vi "PH_ImageCalibrator.read calibration data.vi"(2 "Calibration Data File":path, 5 "error in (no error)":errorcluster) -> (17 "Calibration data":T1, 19 "error out":errorcluster)   [LabVIEW 2014, in "PH_ImageCalibrator.lvlib"]
doc: "This VI reads out the calibration data file. If error in shows an error, the error is passing throung and nothing is done. If there is no incoming error, but an error ocours opening the file, reading the file or unpacking the data, error out is cleaned and the calibration data array is set to be empty. Otherwise the data are given out at the Calibration data cluster."
uses:
  PH_ImageCalibrator.lvlib
  PH_ImageCalibrator.Calibration Data.ctl
  PH_ImageCalibrator.Calibration Data - Version 1.ctl
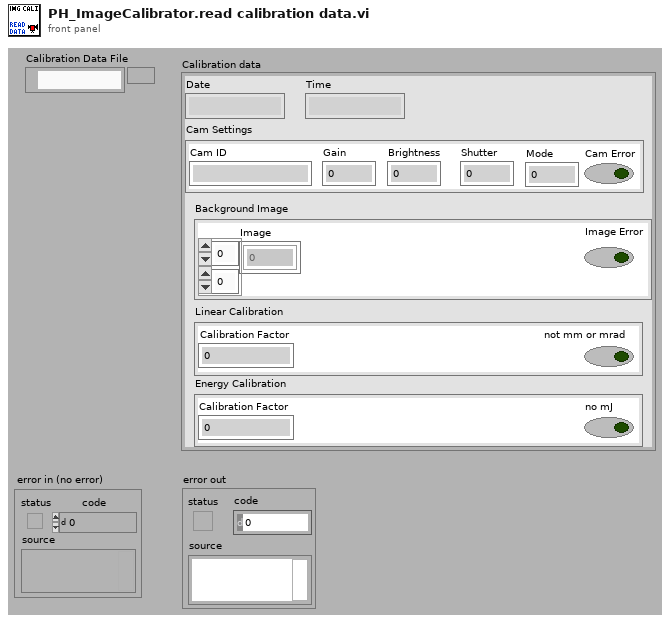
[diagram p1: front panel]
types:
  T1 = typedef "PH_ImageCalibrator.lvlib/PH_ImageCalibrator.Calibration Data.ctl" = cluster{"Date":string, "Time":string, "Cam Settings":cluster{"Cam ID":string, "Gain":dbl, "Brightness":dbl, "Shutter":dbl, "Cam Error":bool, "Mode":i32}, "Background Image":cluster{"Image":dbl[][], "Image Error":bool}, "Linear Calibration":cluster{"Calibration Factor":dbl, "not mm or mrad":bool}, "Energy Calibration":cluster{"Calibration Factor":dbl, "no mJ":bool}}
  T2 = typedef "PH_ImageCalibrator.lvlib/PH_ImageCalibrator.Calibration Data - Version 1.ctl" = cluster{"Date":string, "Time":string, "Cam Settings":cluster{"Serial Number":dbl, "Gain":i32, "Brightness":i32, "Shutter":i32, "Cam Error":bool, "Mode":i32}, "Background Image":cluster{"Image":dbl[][], "Image Error":bool}, "Linear Calibration":cluster{"Calibration Factor":dbl, "not mm or mrad":bool}, "Energy Calibration":cluster{"Calibration Factor":dbl, "no mJ":bool}}
  T3 = cluster{"Calibration Factor":dbl, "not mm or mrad":bool}
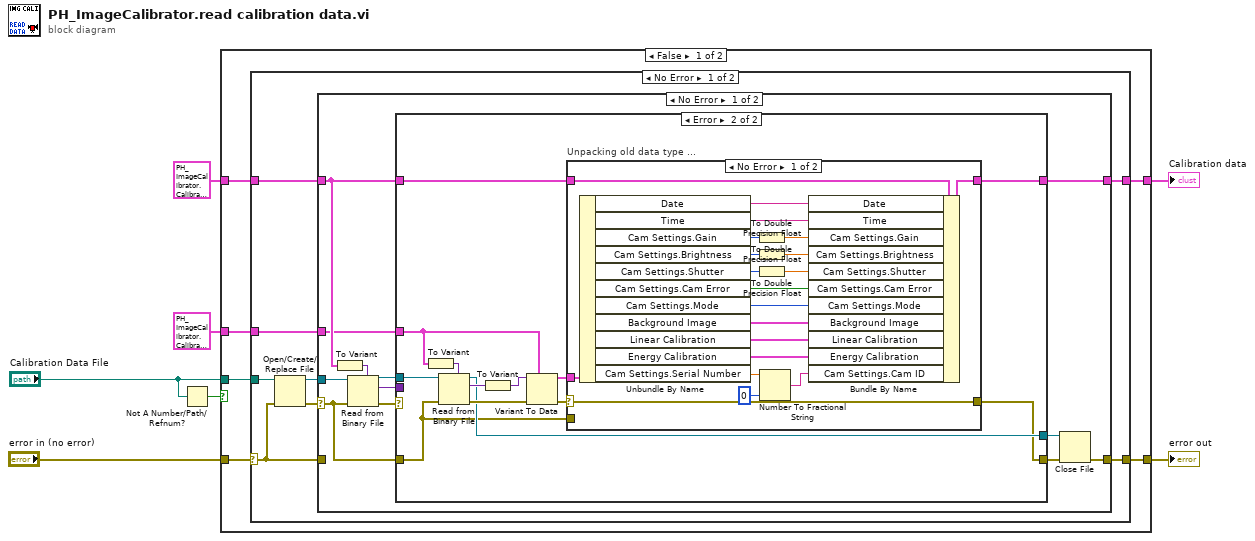
[diagram p0: block diagram]
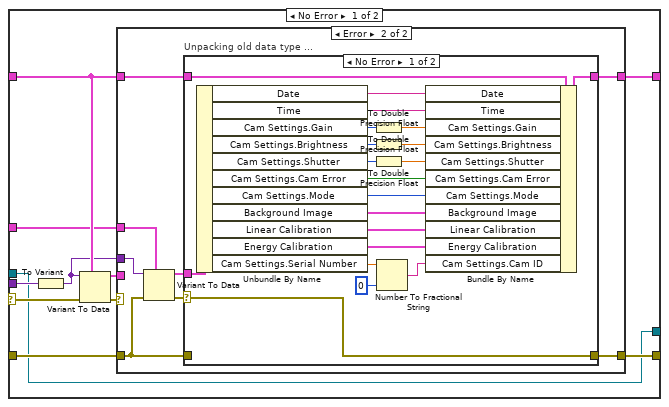
[diagram p2: hidden frame]
diagram:
  n1 = Not A Number/Path/Refnum?(number/path/refnum="Calibration Data File") -> (NaN/Path/Refnum?=w4:bool)
  n2 = case shown="False" w4 {
    tunnel: [w13 w117] -> w7
    tunnel: "error in (no error)" -> [w12 w117]
    tunnel: T1 {"Date"="", "Time"="", "Cam Settings"={"Cam ID"="", "Gain"=0.0, "Brightness"=0.0, "Shutter"=0.0, "Cam Error"=FALSE, "Mode"=0}, "Background Image"={"Image"=[], "Image Error"=FALSE}, "Linear Calibration"={"Calibration Factor"=0.0, "not mm or mrad"=FALSE}, "Energy Calibration"={"Calibration Factor"=0.0, "no mJ"=FALSE}} ("Calibration data") -> [w11 w116]
    tunnel: [w10 w116] -> w5
    tunnel: "Calibration Data File" -> [w9 _]
    tunnel: T2 {"Date"="", "Time"="", "Cam Settings"={"Serial Number"=0.0, "Gain"=0, "Brightness"=0, "Shutter"=0, "Cam Error"=FALSE, "Mode"=0}, "Background Image"={"Image"=[], "Image Error"=FALSE}, "Linear Calibration"={"Calibration Factor"=0.0, "not mm or mrad"=FALSE}, "Energy Calibration"={"Calibration Factor"=0.0, "no mJ"=FALSE}} ("Calibration data - Version 1") -> [w8 _]
    frame False {
      n3 = case shown="No Error" w12 {
        selector: w12 -> [w16 w115]
        tunnel: w9 -> [w20 _]
        tunnel: [w19 w115] -> w13
        tunnel: [w18 w114] -> w10
        tunnel: w11 -> [w15 w114]
        tunnel: w8 -> [w14 _]
        frame No Error {
          n4 = Open/Create/Replace File(file path (use dialog)=w20, error in=w16) -> (refnum out=w21:refnum<file>, error out=w17:errorcluster)  [unwired: 4 in, 1 out]
          n5 = case shown="No Error" w17 {
            selector: w17 -> [w26 _]
            tunnel: w21 -> [w33 _]
            tunnel: [w25 w113] -> w19
            tunnel: [w29 w112] -> w18
            tunnel: w15 -> [w30 w112]
            tunnel: w16 -> [_ w113]
            tunnel: w14 -> [w27 _]
            frame No Error {
              n6 = To Variant(anything=w30) -> (Variant=w31:variant)
              n7 = Read from Binary File(5:w31, 8:w26, 11:w33) -> (0:w28:errorcluster, 2:w32:variant, 3:w23:refnum<file>)  [unwired: 3 in, 1 out]
              n8 = case shown="Error" w28 {
                selector: w28 -> [w38 _]
                tunnel: w32 -> [w44 _]
                tunnel: w30 -> [w42 w78]
                tunnel: [w41 w79] -> w29
                tunnel: [w39 w81] -> w24
                tunnel: w26 -> [w37 w80]
                tunnel: w27 -> [w34 w85]
                tunnel: w23 -> [w36 w84]
                tunnel: [w36 w83] -> w22
                frame No Error {
                  n9 = To Variant(anything=w44) -> (Variant=w35:variant)
                  n10 = Variant To Data(error in=w38, type=w42, Variant=w35) -> (data=w40:T1, error out=w43:errorcluster)
                  n11 = case shown="Error" w43 {
                    selector: w43 -> [w45 _]
                    tunnel: w42 -> [_ w49]
                    tunnel: [w46 w48] -> w41
                    tunnel: w40 -> [w46 _]
                    tunnel: [w45 w47] -> w39
                    tunnel: w37 -> [_ w50]
                    tunnel: w35 -> [_ w54]
                    tunnel: w34 -> [_ w53]
                    frame No Error {
                    }
                    frame Error {
                      n12 = Variant To Data(error in=w50, type=w53, Variant=w54) -> (data=w51:T2, error out=w52:errorcluster)
                      n13 = case "Unpacking old data type ..." shown="No Error" w52 {
                        selector: w52 -> [w74 _]
                        tunnel: [w74 w76] -> w47
                        tunnel: w50 -> [_ w76]
                        tunnel: [w72 w75] -> w48
                        tunnel: w49 -> [w73 w75]
                        tunnel: w51 -> [w71 _]
                        frame No Error {
                          n14 = Unbundle By Name(w71) -> ("Date"=w70:string, "Time"=w65:string, "Cam Settings.Gain"=w61:i32, "Cam Settings.Brightness"=w62:i32, "Cam Settings.Shutter"=w63:i32, "Cam Settings.Cam Error"=w64:bool, "Cam Settings.Mode"=w66:i32, "Background Image"=w67:cluster{"Image":dbl[][], "Image Error":bool}, "Linear Calibration"=w68:T3, "Energy Calibration"=w69:cluster{"Calibration Factor":dbl, "no mJ":bool}, "Cam Settings.Serial Number"=w57:dbl)
                          n15 = To Double Precision Float(number=w61) -> (double precision float=w60:dbl)
                          n16 = To Double Precision Float(number=w62) -> (double precision float=w59:dbl)
                          n17 = To Double Precision Float(number=w63) -> (double precision float=w58:dbl)
                          n18 = Number To Fractional String(number=w57, precision (6)=i16 0) -> (F-format string=w56:string)  [unwired: 2 in]
                          n19 = Bundle By Name(cluster=w73, "Date"=w70, "Time"=w65, "Cam Settings.Gain"=w60, "Cam Settings.Brightness"=w59, "Cam Settings.Shutter"=w58, "Cam Settings.Cam Error"=w64, "Cam Settings.Mode"=w66, "Background Image"=w67, "Linear Calibration"=w68, "Energy Calibration"=w69, "Cam Settings.Cam ID"=w56) -> (w72:T1)
                        }
                        frame Error {
                        }
                      }
                    }
                  }
                }
                frame Error {
                  n20 = To Variant(anything=w85) -> (Variant=w88:variant)
                  n21 = Read from Binary File(5:w88, 8:w80, 11:w84) -> (0:w89:errorcluster, 2:w86:variant, 3:w83:refnum<file>)  [unwired: 3 in, 1 out]
                  n22 = To Variant(anything=w86) -> (Variant=w87:variant)
                  n23 = Variant To Data(error in=w89, type=w85, Variant=w87) -> (data=w77:T2, error out=w82:errorcluster)
                  n24 = case "Unpacking old data type ..." shown="No Error" w82 {
                    selector: w82 -> [w109 _]
                    tunnel: [w109 w111] -> w81
                    tunnel: w80 -> [_ w111]
                    tunnel: [w107 w110] -> w79
                    tunnel: w78 -> [w108 w110]
                    tunnel: w77 -> [w106 _]
                    frame No Error {
                      n25 = Unbundle By Name(w106) -> ("Date"=w105:string, "Time"=w100:string, "Cam Settings.Gain"=w96:i32, "Cam Settings.Brightness"=w97:i32, "Cam Settings.Shutter"=w98:i32, "Cam Settings.Cam Error"=w99:bool, "Cam Settings.Mode"=w101:i32, "Background Image"=w102:cluster{"Image":dbl[][], "Image Error":bool}, "Linear Calibration"=w103:T3, "Energy Calibration"=w104:cluster{"Calibration Factor":dbl, "no mJ":bool}, "Cam Settings.Serial Number"=w92:dbl)
                      n26 = To Double Precision Float(number=w96) -> (double precision float=w95:dbl)
                      n27 = To Double Precision Float(number=w97) -> (double precision float=w94:dbl)
                      n28 = To Double Precision Float(number=w98) -> (double precision float=w93:dbl)
                      n29 = Number To Fractional String(number=w92, precision (6)=i16 0) -> (F-format string=w91:string)  [unwired: 2 in]
                      n30 = Bundle By Name(cluster=w108, "Date"=w105, "Time"=w100, "Cam Settings.Gain"=w95, "Cam Settings.Brightness"=w94, "Cam Settings.Shutter"=w93, "Cam Settings.Cam Error"=w99, "Cam Settings.Mode"=w101, "Background Image"=w102, "Linear Calibration"=w103, "Energy Calibration"=w104, "Cam Settings.Cam ID"=w91) -> (w107:T1)
                    }
                    frame Error {
                    }
                  }
                }
              }
              n31 = Close File(refnum=w22, error in=w24) -> (error out=w25:errorcluster)  [unwired: 1 out]
            }
            frame Error {
            }
          }
        }
        frame Error {
        }
      }
    }
    frame True {
    }
  }
  "error out" <- w7
  "Calibration data" <- w5
